vi "Get Motors.vi"(8 "error in (no error)":errorcluster, 11 "KUKA youBot gripper in":refnum<class "NI_Robotics_KUKA youBot Gripper.lvclass">) -> (0 "error out":errorcluster, 2 "motors":refnum<class "NI_Robotics_KUKA youBot Gripper Motor.lvclass">[](array[class]), 3 "KUKA youBot gripper out":refnum<class "NI_Robotics_KUKA youBot Gripper.lvclass">)   [LabVIEW 2017, in "NI_Robotics_KUKA youBot Host.lvlib" / "NI_Robotics_KUKA youBot Gripper.lvclass"]
uses:
  <vilib>/robotics/KUKA youBot/Basic Device/Gripper/NI_Robotics_KUKA youBot Gripper.lvclass
  <vilib>/robotics/KUKA youBot/Motor/Gripper Motor/NI_Robotics_KUKA youBot Gripper Motor.lvclass
  <vilib>/robotics/KUKA youBot/Basic Device/Gripper/NI_Robotics_KUKA youBot Gripper.lvclass/NI_Robotics_KUKA youBot Gripper.ctl
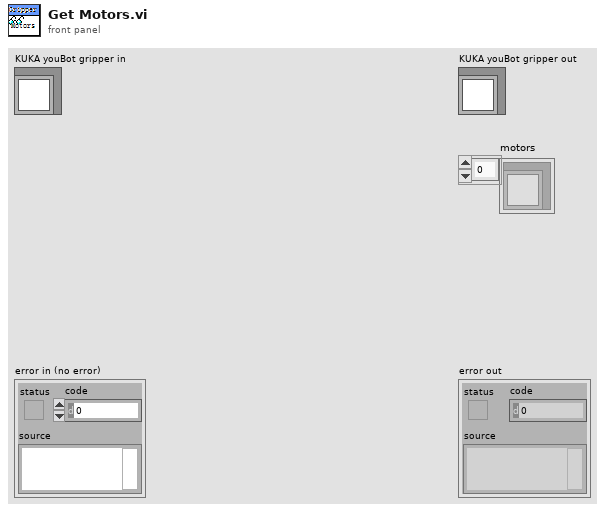
[diagram p1: front panel]
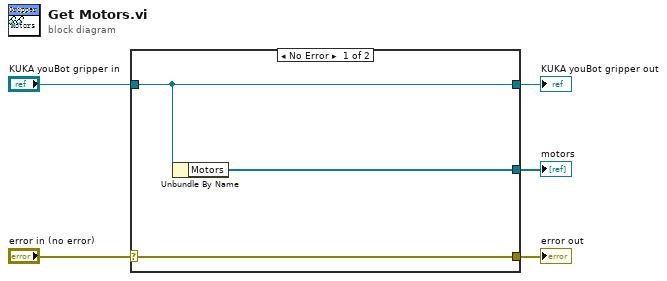
[diagram p0: block diagram]
diagram:
  n1 = case shown="No Error" "error in (no error)" {
    selector: "error in (no error)" -> [w8 w9]
    tunnel: [w8 w9] -> w4
    tunnel: [w7 w10] -> w2
    tunnel: "KUKA youBot gripper in" -> [w7 w10]
    tunnel: [w6 _] -> w1
    frame No Error {
      n2 = Unbundle By Name(w7) -> ("Motors"=w6:refnum<class "NI_Robotics_KUKA youBot Gripper Motor.lvclass">[])
    }
    frame Error {
    }
  }
  "error out" <- w4
  "KUKA youBot gripper out" <- w2
  "motors" <- w1
